vi "Establish Connection - Server.vi"(3 "error in (no error)":errorcluster) -> (7 "Connection Info":T1, 10 "error out":errorcluster)   [LabVIEW 2020]
doc: "Tests ports in direction of cliend to server"
panel:
  in  "Message to Send":string="You are currently accessing TCP Named Service - Server.vi from client %s on port %d."
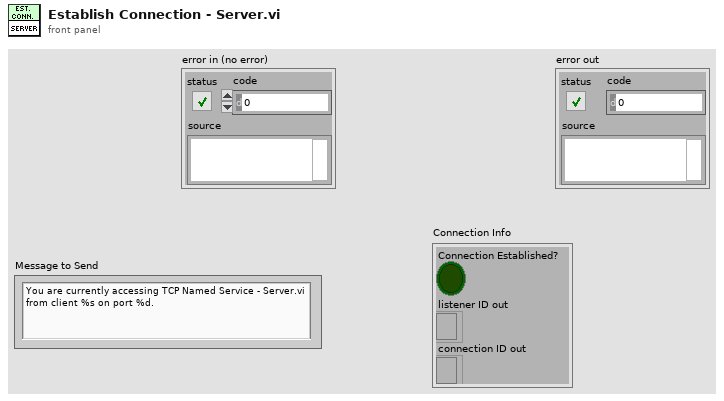
[diagram p1: front panel]
types:
  T1 = cluster{"Connection Established?":bool, "listener ID out":refnum<k5>, "connection ID out":refnum<k5>}
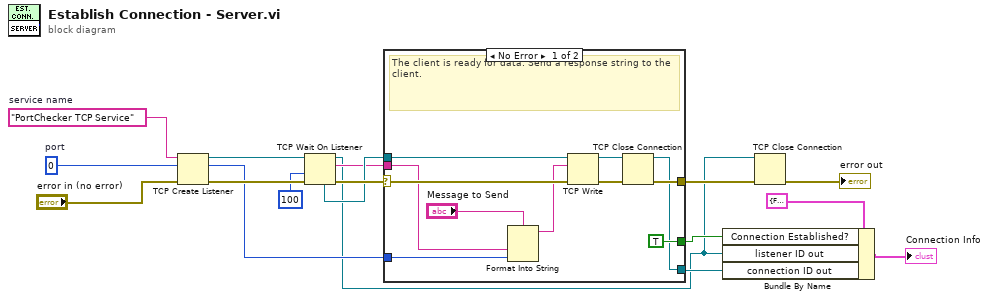
[diagram p0: block diagram]
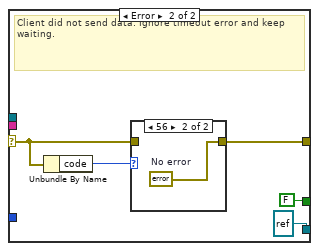
[diagram p2: hidden frame]
diagram:
  w14 = u16 0  # port
  w13 = "PortChecker TCP Service"  # service name
  n1 = TCP Create Listener(8:"error in (no error)", 10:w14, 11:w13) -> (0:w16:errorcluster, 2:w15:u16, 3:w17:refnum<k5>)  [unwired: 2 in]
  n2 = TCP Wait On Listener(8:w16, 9:100 ("timeout ms (25000)"), 11:w17) -> (0:w11:errorcluster, 2:w8:string, 3:w1:refnum<k5>, 4:w10:refnum<k5>)  [unwired: 1 in, 1 out]
  n3 = case shown="No Error" w11 {
    selector: w11 -> [w28 w33]
    tunnel: [w21 w31] -> w2
    tunnel: w10 -> [w22 _]
    tunnel: w15 -> [w26 _]
    tunnel: w8 -> [w24 _]
    tunnel: [TRUE FALSE] -> w6
    tunnel: [w18 refnum<k5> refnum ("listener ID")] -> w5
    frame No Error {
      # "The client is ready for data. Send a response string to the client."
      n4 = Format Into String(format string="Message to Send", w24, w26) -> (resulting string=w23:string)  [unwired: 2 in, 1 out]
      n5 = TCP Write(connection ID=w22, data in=w23, error in (no error)=w28) -> (connection ID out=w20:refnum<k5>, error out=w27:errorcluster)  [unwired: 1 in, 1 out]
      n6 = TCP Close Connection(connection ID=w20, error in (no error)=w27) -> (connection ID out=w18:refnum<k5>, error out=w21:errorcluster)  [unwired: 1 in]
    }
    frame Error {
      # "Client did not send data. Ignore timeout error and keep waiting."
      n7 = Unbundle By Name(w33) -> ("code"=w32:i32)
      n8 = case shown="56" w32 {
        tunnel: w33 -> [w34 _]
        tunnel: [w34 w35] -> w31
        frame Default {
        }
        frame 56 {
          w35 = errorcluster {"status"=FALSE, "code"=0, "source"=""}  # No error
        }
      }
    }
  }
  n9 = Bundle By Name(cluster=T1 {"Connection Established?"=FALSE, "listener ID out"=refnum, "connection ID out"=refnum} ("Connection Info"), "Connection Established?"=w6, "listener ID out"=w1, "connection ID out"=w5) -> (→"Connection Info":T1)
  n10 = TCP Close Connection(connection ID=w1, error in (no error)=w2) -> (error out=→"error out":errorcluster)  [unwired: 1 in, 1 out]
